vi "get refnums.vi"(8 "error in (no error)":errorcluster, 11 "Elevator in":refnum<class "Elevator.lvclass">) -> (0 "error out":errorcluster, 1 "motor refnums":T1, 3 "Elevator out":refnum<class "Elevator.lvclass">)   [LabVIEW 2018, in "Elevator.lvlib" / "Elevator.lvclass"]
doc: "This VI does nothing."
uses:
  Elevator.lvclass
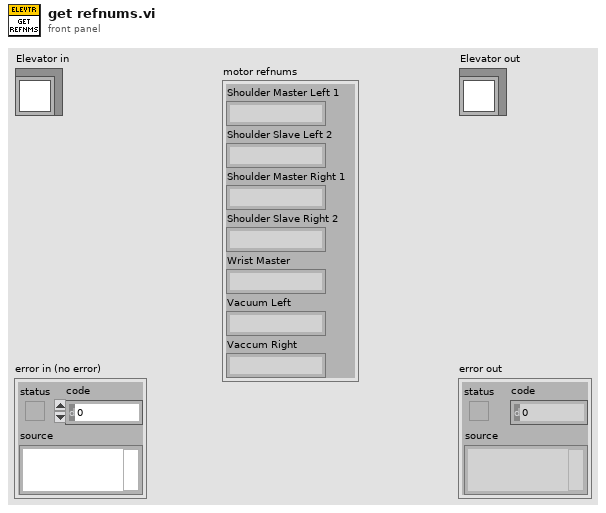
[diagram p1: front panel]
types:
  T1 = cluster{"Shoulder Master Left 1":string, "Shoulder Slave Left 2":string, "Shoulder Master Right 1":string, "Shoulder Slave Right 2 ":string, "Wrist Master ":string, "Vacuum Left":string, "Vaccum Right":string}
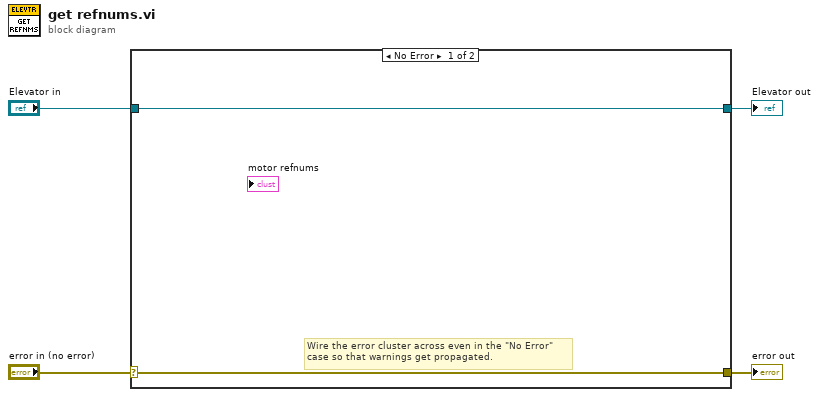
[diagram p0: block diagram]
diagram:
  n1 = case shown="No Error" "error in (no error)" {
    selector: "error in (no error)" -> [w5 w8]
    tunnel: [w5 w8] -> w3
    tunnel: [w6 w7] -> w1
    tunnel: "Elevator in" -> [w6 w7]
    frame No Error {
      # "Wire the error cluster across even in the \"No Error\"\ncase so that warnings get propagated."
    }
    frame Error {
    }
  }
  "error out" <- w3
  "Elevator out" <- w1
